vi "ReplaesDotOrComm (SubVI).vi"(6 "comm?":bool, 9 "NewVal":string[][](array[string]), 11 "OldVal":string[][](array[string])) -> (1 "output array":string[][](array[string]))   [LabVIEW 2017]
panel:
  out "i":i32
  out "element":string
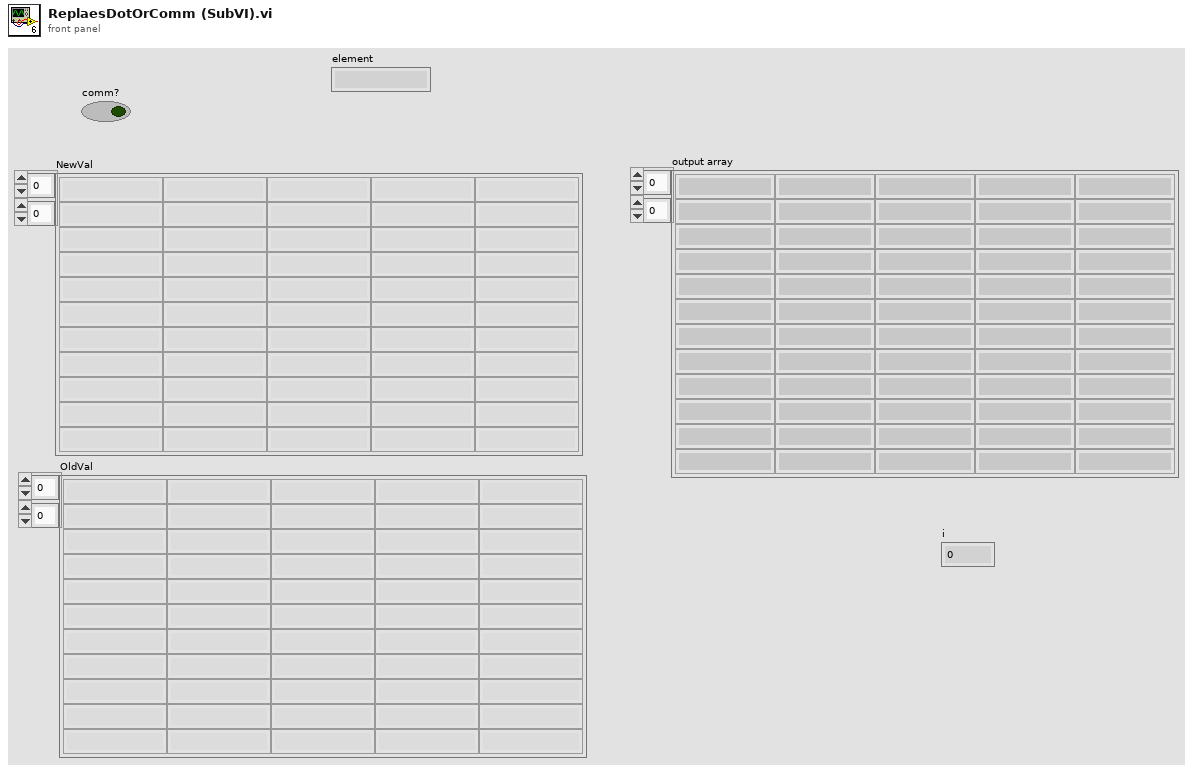
[diagram p1: front panel]
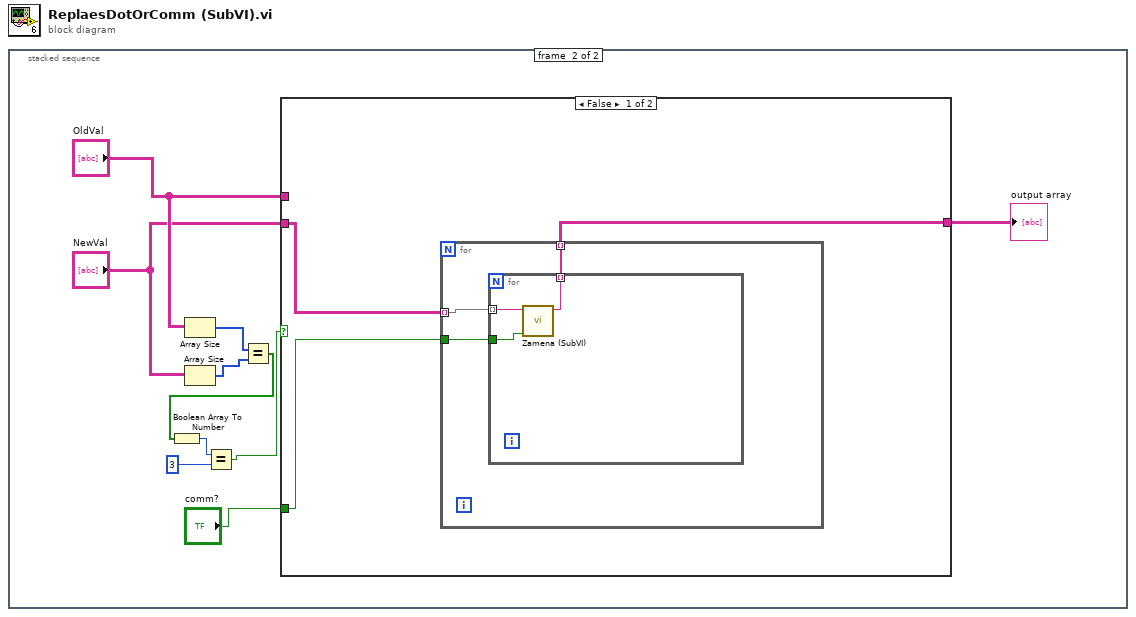
[diagram p0: block diagram]
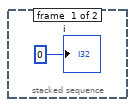
[diagram p2: hidden frame]
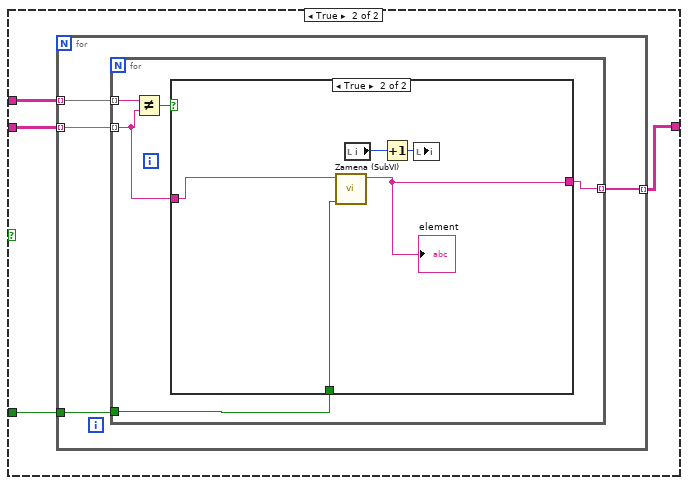
[diagram p3: hidden frame]
diagram:
  n1 = stacked-sequence {
    frame #0 {
      "i" <- 0 ("i")
    }
    frame #1 {
      n2 = Array Size(array="OldVal") -> (size(s)=w8:i32[])
      n3 = Array Size(array="NewVal") -> (size(s)=w7:i32[])
      n4 = Equal?(x=w8, y=w7) -> (x = y?=w6:bool[])
      n5 = Boolean Array To Number(Boolean array=w6) -> (number=w5:u32)
      n6 = Equal?(x=w5, y=u32 3) -> (x = y?=w3:bool)
      n7 = case shown="False" w3 {
        tunnel: [w12 w24] -> w11
        tunnel: "OldVal" -> [_ w23]
        tunnel: "NewVal" -> [w14 w22]
        tunnel: "comm?" -> [w13 w21]
        frame False {
          n8 = for {
            tunnel: w14 -> [w17] mode=indexing
            tunnel: w13 -> [w16]
            tunnel: [w15] -> w12 mode=indexing
            n9 = for {
              tunnel: w17 -> [w20] mode=indexing
              tunnel: w16 -> [w19]
              tunnel: [w18] -> w15 mode=indexing
              n10 = call "Zamena (SubVI).vi"("comm?"=w19, "input string"=w20) -> ("result string 2"=w18:string)  [unwired: 9 in]
            }
          }
        }
        frame True {
          n11 = for {
            tunnel: w23 -> [w28] mode=indexing
            tunnel: w22 -> [w27] mode=indexing
            tunnel: [w26] -> w24 mode=indexing
            tunnel: w21 -> [w25]
            n12 = for {
              tunnel: w28 -> [w33] mode=indexing
              tunnel: w27 -> [w31] mode=indexing
              tunnel: [w30] -> w26 mode=indexing
              tunnel: w25 -> [w29]
              n13 = Not Equal?(x=w33, y=w31) -> (x != y?=w32:bool)
              n14 = case shown="True" w32 {
                tunnel: w31 -> [w34 w39]
                tunnel: [w34 w38] -> w30
                tunnel: w29 -> [_ w35]
                frame False {
                }
                frame True {
                  n15 = call "Zamena (SubVI).vi"("comm?"=w35, "input string"=w39) -> ("result string 2"=w38:string)  [unwired: 9 in]
                  "element" <- w38
                  n16 = local read "i"() -> (w37:i32)
                  n17 = Increment(x=w37) -> (x+1=w36:i32)
                  n18 = local write "i"(w36) -> ()
                }
              }
            }
          }
        }
      }
      "output array" <- w11
    }
  }
